vi "ex 1 - clock.vi"() -> ()   [LabVIEW 2016]
panel:
  out "Gauge":dbl(knob) scale=0.0..60.0
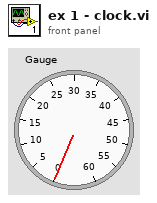
[diagram p1: front panel]
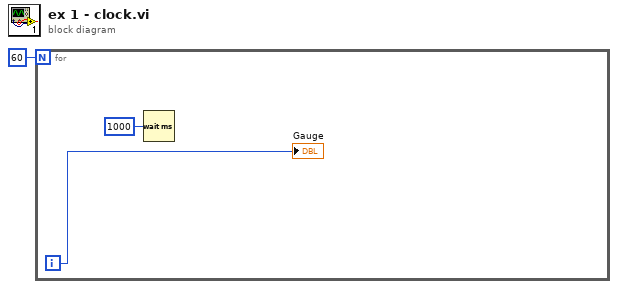
[diagram p0: block diagram]
diagram:
  n1 = for {
    N: 60 -> [_]
    i -> [w2]
    n2 = Wait (ms)(milliseconds to wait=u32 1000) -> ()  [unwired: 1 out]
    "Gauge" <- w2
  }
